vi "ReportVelocityStateDecode.vi"(1 "Payload":string) -> (0 "VelocityState":T1)   [LabVIEW 2009]
uses:
  Support Files/VelocityState.ctl
  Support Files/TimeRec.ctl
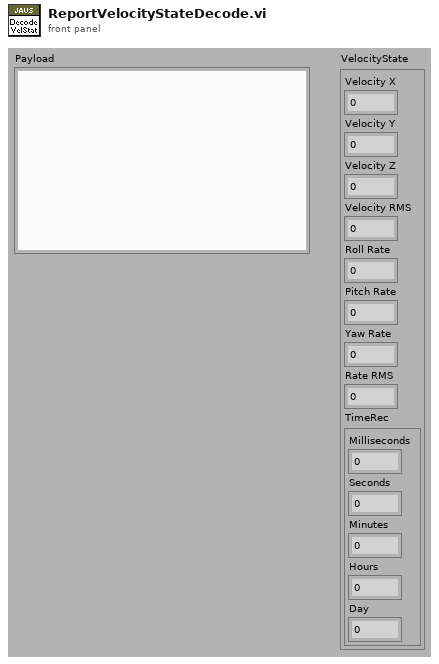
[diagram p1: front panel]
types:
  T1 = typedef "VelocityState.ctl" = cluster{"Velocity X":dbl, "Velocity Y":dbl, "Velocity Z":dbl, "Velocity RMS":dbl, "Roll Rate":dbl, "Pitch Rate":dbl, "Yaw Rate":dbl, "Rate RMS":dbl, "TimeRec":T2}
  T2 = typedef "TimeRec.ctl" = cluster{"Milliseconds":u32, "Seconds":u32, "Minutes":u32, "Hours":u32, "Day":u32}
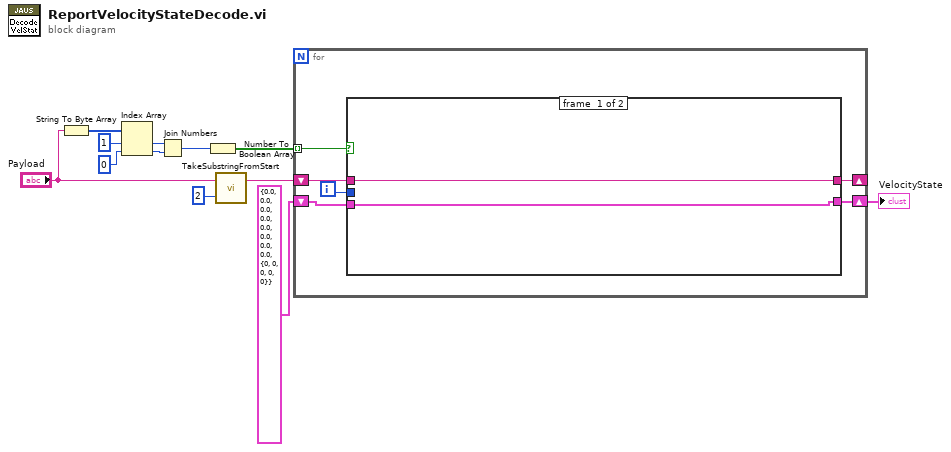
[diagram p0: block diagram]
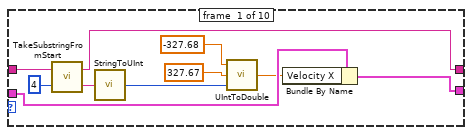
[diagram p3: hidden frame]
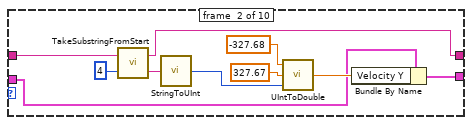
[diagram p4: hidden frame]
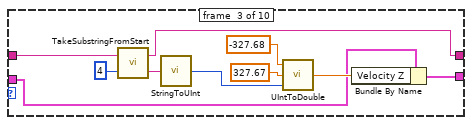
[diagram p5: hidden frame]
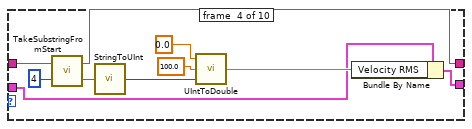
[diagram p6: hidden frame]
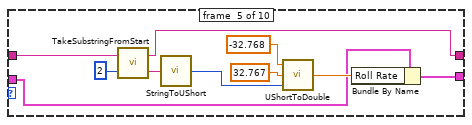
[diagram p7: hidden frame]
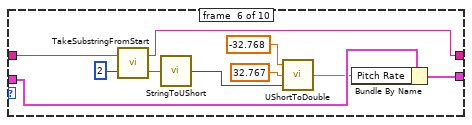
[diagram p8: hidden frame]
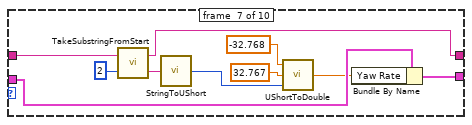
[diagram p9: hidden frame]
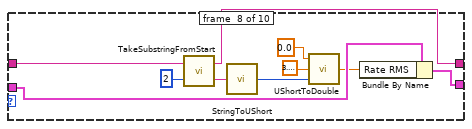
[diagram p10: hidden frame]
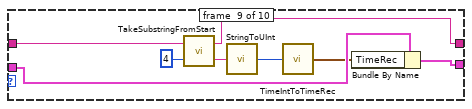
[diagram p11: hidden frame]
diagram:
  n1 = String To Byte Array(string="Payload") -> (unsigned byte array=w4:u8[])
  n2 = Index Array(array=w4, index #1=1 ("index"), index #2=0 ("index")) -> (element #1=w8:u8, element #2=w6:u8)
  n3 = Join Numbers(hi=w8, lo=w6) -> ((hi.lo)=w5:u16)
  n4 = Number To Boolean Array(number=w5) -> (Boolean array=w7:bool[])
  n5 = call "TakeSubstringFromStart.vi"("offset"=2, "string"="Payload") -> ("string after offset"=w1:string)  [unwired: 1 out]
  n6 = for {
    tunnel: w7 -> [w18] mode=indexing
    shift-right: [w15] -> w10
    shift-left: T1 {"Velocity X"=0.0, "Velocity Y"=0.0, "Velocity Z"=0.0, "Velocity RMS"=0.0, "Roll Rate"=0.0, "Pitch Rate"=0.0, "Yaw Rate"=0.0, "Rate RMS"=0.0, "TimeRec"={"Milliseconds"=0, "Seconds"=0, "Minutes"=0, "Hours"=0, "Day"=0}} ("VelocityState") -> [w16]
    shift-right: [w13] -> _
    shift-left: w1 -> [w14]
    i -> [w17]
    n7 = case shown="False" w18 {
      tunnel: w17 -> [_ w25]
      tunnel: w16 -> [w20 w24]
      tunnel: [w20 w23] -> w15
      tunnel: w14 -> [w19 w22]
      tunnel: [w19 w21] -> w13
      frame #0 {
      }
      frame #1 {
        n8 = case shown="3" w25 {
          tunnel: w24 -> [w35 w42 w52 w62 w72 w84 w94 w104 w113 w114]
          tunnel: [w26 w41 w51 w61 w71 w85 w95 w105 w112 w114] -> w23
          tunnel: w22 -> [w31 w39 w48 w58 w69 w79 w89 w98 w108 w115]
          tunnel: [w29 w37 w47 w56 w66 w76 w87 w96 w106 w115] -> w21
          frame #0 {
            n9 = call "TakeSubstringFromStart.vi"("offset"=4, "string"=w31) -> ("string before offset"=w28:string, "string after offset"=w29:string)
            n10 = call "StringToUInt.vi"("string"=w28) -> ("UInt"=w27:u32)
            n11 = call "UIntToDouble.vi"("Value"=w27, "Max"=327.67 ("Min"), "Min"=-327.68) -> ("Number"=w32:dbl)
            n12 = Bundle By Name(cluster=w35, "Velocity X"=w32) -> (w26:T1)
          }
          frame #1 {
            n13 = call "TakeSubstringFromStart.vi"("offset"=4, "string"=w39) -> ("string before offset"=w40:string, "string after offset"=w37:string)
            n14 = call "StringToUInt.vi"("string"=w40) -> ("UInt"=w36:u32)
            n15 = call "UIntToDouble.vi"("Value"=w36, "Max"=327.67 ("Min"), "Min"=-327.68) -> ("Number"=w43:dbl)
            n16 = Bundle By Name(cluster=w42, "Velocity Y"=w43) -> (w41:T1)
          }
          frame #2 {
            n17 = call "TakeSubstringFromStart.vi"("offset"=4, "string"=w48) -> ("string before offset"=w50:string, "string after offset"=w47:string)
            n18 = call "StringToUInt.vi"("string"=w50) -> ("UInt"=w46:u32)
            n19 = call "UIntToDouble.vi"("Value"=w46, "Max"=327.67 ("Min"), "Min"=-327.68) -> ("Number"=w53:dbl)
            n20 = Bundle By Name(cluster=w52, "Velocity Z"=w53) -> (w51:T1)
          }
          frame #3 {
            n21 = call "TakeSubstringFromStart.vi"("offset"=4, "string"=w58) -> ("string before offset"=w60:string, "string after offset"=w56:string)
            n22 = call "StringToUInt.vi"("string"=w60) -> ("UInt"=w57:u32)
            n23 = call "UIntToDouble.vi"("Value"=w57, "Max"=100.0 ("Min"), "Min"=0.0) -> ("Number"=w63:dbl)
            n24 = Bundle By Name(cluster=w62, "Velocity RMS"=w63) -> (w61:T1)
          }
          frame #4 {
            n25 = call "TakeSubstringFromStart.vi"("offset"=2, "string"=w69) -> ("string before offset"=w68:string, "string after offset"=w66:string)
            n26 = call "StringToUShort.vi"("string"=w68) -> ("UShort"=w67:u16)
            n27 = call "UShortToDouble.vi"("Value"=w67, "Max"=32.767 ("Min"), "Min"=-32.768) -> ("Number"=w73:dbl)
            n28 = Bundle By Name(cluster=w72, "Roll Rate"=w73) -> (w71:T1)
          }
          frame #5 {
            n29 = call "TakeSubstringFromStart.vi"("offset"=2, "string"=w79) -> ("string before offset"=w78:string, "string after offset"=w76:string)
            n30 = call "StringToUShort.vi"("string"=w78) -> ("UShort"=w77:u16)
            n31 = call "UShortToDouble.vi"("Value"=w77, "Max"=32.767 ("Min"), "Min"=-32.768) -> ("Number"=w81:dbl)
            n32 = Bundle By Name(cluster=w84, "Pitch Rate"=w81) -> (w85:T1)
          }
          frame #6 {
            n33 = call "TakeSubstringFromStart.vi"("offset"=2, "string"=w89) -> ("string before offset"=w88:string, "string after offset"=w87:string)
            n34 = call "StringToUShort.vi"("string"=w88) -> ("UShort"=w86:u16)
            n35 = call "UShortToDouble.vi"("Value"=w86, "Max"=32.767 ("Min"), "Min"=-32.768) -> ("Number"=w91:dbl)
            n36 = Bundle By Name(cluster=w94, "Yaw Rate"=w91) -> (w95:T1)
          }
          frame #7 {
            n37 = call "TakeSubstringFromStart.vi"("offset"=2, "string"=w98) -> ("string before offset"=w99:string, "string after offset"=w96:string)
            n38 = call "StringToUShort.vi"("string"=w99) -> ("UShort"=w97:u16)
            n39 = call "UShortToDouble.vi"("Value"=w97, "Max"=3.141592653589793 ("Min"), "Min"=0.0) -> ("Number"=w101:dbl)
            n40 = Bundle By Name(cluster=w104, "Rate RMS"=w101) -> (w105:T1)
          }
          frame #8 {
            n41 = call "TakeSubstringFromStart.vi"("offset"=4, "string"=w108) -> ("string before offset"=w110:string, "string after offset"=w106:string)
            n42 = call "StringToUInt.vi"("string"=w110) -> ("UInt"=w107:u32)
            n43 = call "TimeIntToTimeRec.vi"("Time Int"=w107) -> ("TimeRec"=w111:T2)
            n44 = Bundle By Name(cluster=w113, "TimeRec"=w111) -> (w112:T1)
          }
          frame #9 {
          }
        }
      }
    }
  }
  "VelocityState" <- w10
